vi "GoToSkill.vi"(6 "Position":dbl[](array[numeric]), 8 "error in (no error)":errorcluster, 9 "BallRef":refnum<class "Ball.lvclass">, 10 "Robot in":refnum<class "Robot.lvclass">, 11 "GoToSkill in":refnum<class "GoToSkill.lvclass">) -> (0 "error out":errorcluster, 2 "Robot out":refnum<class "Robot.lvclass">, 3 "GoToSkill out":refnum<class "GoToSkill.lvclass">)   [LabVIEW 2021, in "GoToSkill.lvclass"]
uses:
  GoToSkill.lvclass
  Robot_class/Robot.lvclass
  Ball_class/Ball.lvclass
  Utilities_class/Utilities.lvclass
  Robot_class/Robot.lvclass/Robot.ctl
  Robot_class/Write dest_x.vi
  Robot_class/Write dest_y.vi
  Robot_class/Write dest_orientation.vi
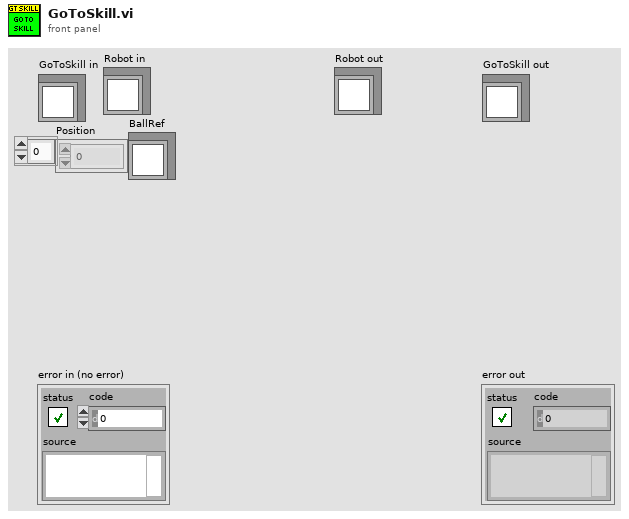
[diagram p1: front panel]
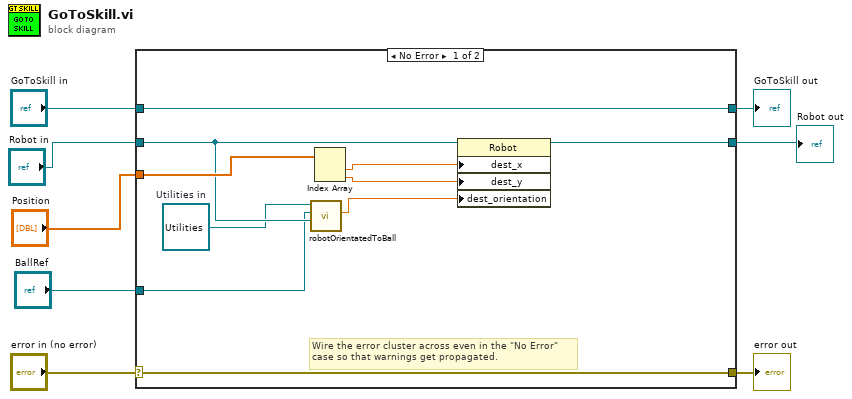
[diagram p0: block diagram]
diagram:
  n1 = case shown="No Error" "error in (no error)" {
    selector: "error in (no error)" -> [w17 w20]
    tunnel: [w17 w20] -> w7
    tunnel: [w18 w19] -> w5
    tunnel: "GoToSkill in" -> [w18 w19]
    tunnel: "Robot in" -> [w11 _]
    tunnel: "Position" -> [w16 _]
    tunnel: [w13 _] -> w2
    tunnel: "BallRef" -> [w9 _]
    frame No Error {
      w10 = refnum<class "Utilities.lvclass"> refnum  # Utilities in
      # "Wire the error cluster across even in the \"No Error\"\ncase so that warnings get propagated."
      n2 = call "robotOrientatedToBall.vi"("Robot"=w11, "BallRef"=w9, "Utilities in"=w10) -> ("Orientation"=w12:dbl)  [unwired: 6 in, 2 out]
      n3 = Index Array(array=w16) -> (element #1=w15:dbl, element #2=w14:dbl)  [unwired: 2 in]
      n4 = property class="Robot"(reference=w11, "dest_x"=w15, "dest_y"=w14, "dest_orientation"=w12) -> (reference out=w13:refnum<class "Robot.lvclass">)  [unwired: 1 in, 1 out]
    }
    frame Error {
    }
  }
  "error out" <- w7
  "GoToSkill out" <- w5
  "Robot out" <- w2
